vi "ziSetValueComplexArray.vi"(3 "Error In":errorcluster, 4 "Values":cdb[](array[numeric]), 5 "Paths":string[](array[string]), 6 "Handle In":T1 {"Handle" format="0x%08x"; "Conn" format="0x%08x"}) -> (0 "Error Out":errorcluster, 2 "Handle Out":T1 {"Handle" format="0x%08x"; "Conn" format="0x%08x"})   [LabVIEW 2018, in "Zurich Instruments LabOne.lvlib"]
doc: "This vi sets values to the nodes specified in Path to Value. More than one node can be set if a wildcard is used in Path. The i-th element of Paths receives the i-th value of Values."
uses:
  Zurich Instruments LabOne.lvlib
  ziTypeHandle.ctl
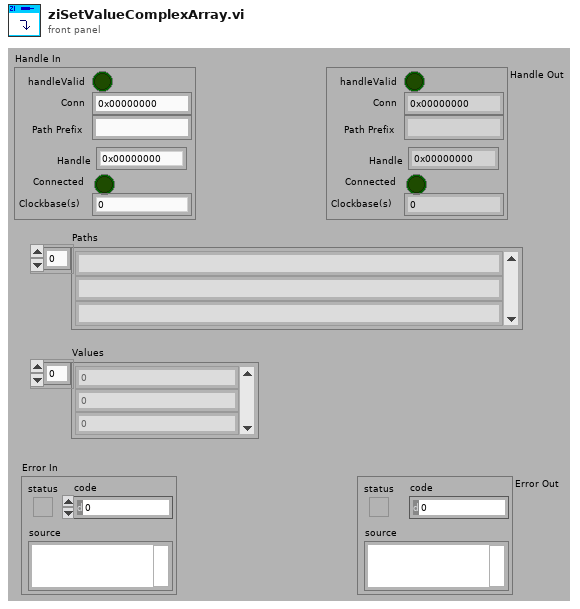
[diagram p1: front panel]
types:
  T1 = typedef "Zurich Instruments LabOne.lvlib/ziTypeHandle.ctl" = cluster{"handleValid":bool, "Conn":u64, "Path Prefix":string, "Handle":u64, "Connected":bool, "Clockbase(s)":dbl}
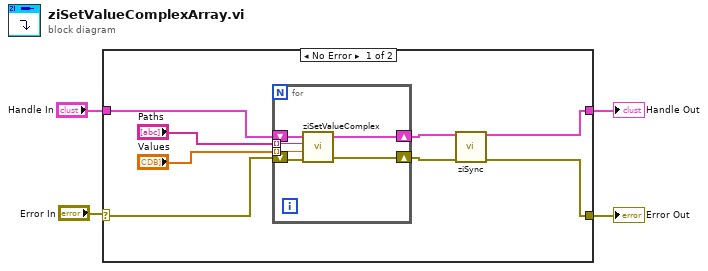
[diagram p0: block diagram]
diagram:
  n1 = case shown="No Error" "Error In" {
    selector: "Error In" -> [w10 w20]
    tunnel: [w5 w20] -> w4
    tunnel: [w6 w19] -> w3
    tunnel: "Handle In" -> [w9 w19]
    frame No Error {
      n2 = for {
        tunnel: "Paths" -> [w18] mode=indexing
        tunnel: "Values" -> [w17] mode=indexing
        shift-right: [w15] -> w8
        shift-left: w10 -> [w16]
        shift-right: [w14] -> w7
        shift-left: w9 -> [w13]
        n3 = call "ziSetValueComplex.vi"("Error In"=w16, "Value"=w17, "Path"=w18, "Handle In"=w13) -> ("Error Out"=w15:errorcluster, "Handle Out"=w14:T1)  [unwired: 1 in]
      }
      n4 = call "ziSync.vi"("Handle In"=w7, "Error In"=w8) -> ("Handle Out"=w6:T1, "Error Out"=w5:errorcluster)  [unwired: 12 in]
    }
    frame Error {
    }
  }
  "Error Out" <- w4
  "Handle Out" <- w3
